vi "_LecturaLOG_Datos_TDMS.vi"(11 "Path":path) -> ()   [LabVIEW 2018]
uses:
  TypeDefsTopside/Top Data.ctl
  Shared/Type Defs/ROV States.ctl
  TypeDefsSubsea/Modos Control.ctl
  TypeDefsTopside/DAQ Top Data.ctl
  TypeDefsTopside/User Data.ctl
  TypeDefsTopside/CI Data.ctl
  TypeDefsTopside/Surface Input Data.ctl
  TypeDefsTopside/Virtual User Interface Data.ctl
  TypeDefsTopside/Top Control.ctl
  TypeDefsSubsea/Sub Data.ctl
  TypeDefsSubsea/Sub Status.ctl
  Shared/Type Defs/SMP.ctl
  Shared/Type Defs/PWR.ctl
  Shared/Type Defs/Motor.ctl
  Shared/Type Defs/MotorNames.ctl
  Shared/Type Defs/SmartCard.ctl
  Shared/Type Defs/Box Names.ctl
  TypeDefsSubsea/Sub Control.ctl
  TypeDefsSubsea/ROV Outputs.ctl
  TypeDefsSubsea/Motor Control.ctl
  TypeDefsSubsea/Type Defs Subsea.lvlib
  TypeDefsTopside/Type Defs Topside.lvlib
panel:
  out "Progreso TopData":i32
  out "Progreso SubData":i32
  out "String":string
  out "subarray":T1[](array[typedef]) {"Control"."motor_ctrl_array"."sensor" format="%#.2f"; "Control"."motor_ctrl_array"."setpoint" format="%#.2f"; "Control"."dac_outputs" format="%#.2f"; "PWR"."motor_array"."motor_name" items=["Motor1", "Motor2", "Motor3", "Motor4", "Motor5", "Motor6"]}
  out "TppData":T14[](array[typedef]) {"Virtual CI"."pot_c2" step=0.1; "Virtual CI"."pot_c1" step=0.01; "Virtual CI"."pot_gen" step=1.0; "Virtual CI"."pot_l3" step=0.01; "Virtual CI"."pot_l2" step=0.01; "Virtual CI"."pot_l1" step=0.01; "Virtual CI"."pot_m6" step=0.01; "Virtual CI"."pot_m5" step=0.01; "Virtual CI"."pot_m4" step=0.01; "Virtual CI"."pot_m3" step=0.01; "Virtual CI"."pot_m2" step=0.01; "Virtual CI"."pot_m1" step=0.01; "DAQ"."vess_ahrs_"."yaw" format="%.2g"; "DAQ"."vess_ahrs_"."roll" format="%.2g"; "DAQ"."vess_ahrs_"."pitch" format="%.2g"; "DAQ"."usbl_"."z" format="%.7g"; "DAQ"."usbl_"."y" format="%.7g"; "DAQ"."usbl_"."x" format="%.7g"; "DAQ"."gps_"."alt" format="%.7g"; "DAQ"."gps_"."lon" format="%.7g"; "DAQ"."gps_"."lat" format="%.7g"}
  in  "index":i32
  out "Waveform Graph":waveform(dbl)[](graph)
  out "Fecha y hora fin":timestamp
  out "Fecha y hora Inicio":timestamp
  out "error out":errorcluster
  out "Total datos":i32
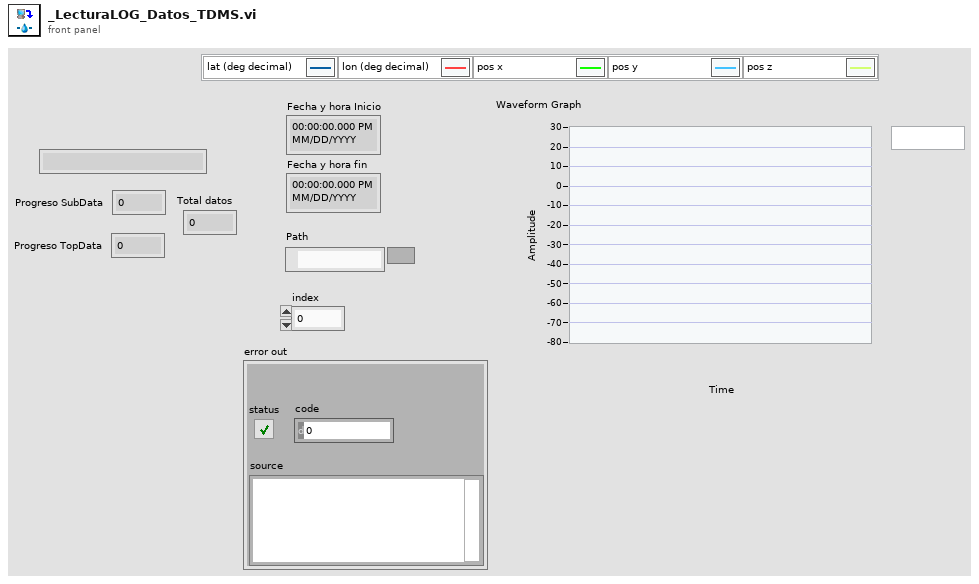
[diagram p1: front panel]
types:
  T1 = typedef "Type Defs Subsea.lvlib/Sub Data.ctl" = cluster{"Status":T2, "AHRS":cluster{"id_sensor":u32, "id_daq":u64, "pitch":dbl, "roll":dbl, "heading":dbl, "accel_x":dbl, "accel_y":dbl, "accel_z":dbl, "gyr_x":dbl, "gyr_y":dbl, "gyr_z":dbl, "mag_x":dbl, "mag_y":dbl, "mag_z":dbl, "acquisition_time":timestamp}, "CTD":cluster{"id_sensor":u32, "id_daq":u64, "pressure":dbl, "temperature":dbl, "conductivity":dbl, "density":dbl, "salinity":dbl, "speed_of_sound":dbl, "depth":dbl, "acquisition_time":timestamp}, "ALTIMETER":cluster{"id_sensor":u32, "id_daq":u64, "altitude":dbl, "acquisition_time":timestamp}, "SMP":T4, "PWR":T5, "SC_PWR":T8, "SC_CPU":T8, "SC_SMP":T8, "Control":T10}
  T2 = typedef "Type Defs Subsea.lvlib/Sub Status.ctl" = cluster{"id_sensor":u32, "id_daq":u32, "sub_ind":bool, "sample_time":i64, "sc_ind":bool[], "rov_states":T3, "acquisition_time":timestamp}
  T3 = typedef "Type Defs Subsea.lvlib/ROV States.ctl" = enum16{"INIT", "IDLE", "TEST", "RUN", "EMERGENCY", "EXIT"}
  T4 = typedef "Type Defs Subsea.lvlib/SMP.ctl" = cluster{"id_sensor":u32, "id_daq":u64, "liquid_smp1":bool, "liquid_smp2":bool, "liquid_smp3":bool, "liquid_smp4":bool, "solid_smp1":bool, "solid_smp2":bool, "supply_12v":bool, "motor_signal1":dbl, "motor_signal2":dbl, "cur_liq_1":dbl, "cur_liq_2":dbl, "acquisition_time":timestamp}
  T5 = typedef "Type Defs Topside.lvlib/PWR.ctl" = cluster{"id_sensor":u32, "id_daq":u64, "ac_status":bool, "voltage_hvdc":dbl, "current_hvdc":dbl, "motor_array":T6[], "light1":dbl, "light2":dbl, "light_sphere":dbl, "voltage_l1_l2":dbl, "voltage_l2_l3":dbl, "voltage_l1_l3":dbl, "current_l1":dbl, "current_l2":dbl, "current_l3":dbl, "current_lights":dbl, "temp_ac_filter":dbl, "acquisition_time":timestamp}
  T6 = typedef "Type Defs Subsea.lvlib/Motor.ctl" = cluster{"motor_name":T7, "status":bool, "ctrl_signal":dbl, "current":dbl, "speed":dbl}
  T7 = typedef "Type Defs Subsea.lvlib/MotorNames.ctl" = u16
  T8 = typedef "Type Defs Subsea.lvlib/SmartCard.ctl" = cluster{"id_sensor":u32, "id_daq":u64, "box_name":T9, "mode":enum16{"OFF", "STANDBY", "TESTING", "RUN", "EMERGENCY"}, "stat":dbl, "lps":dbl, "controller":dbl, "voltage":dbl, "current":dbl, "temperature":dbl, "humidity":dbl, "leak":dbl, "pressure":dbl, "acquisition_time":timestamp}
  T9 = typedef "Type Defs Subsea.lvlib/Box Names.ctl" = enum16{"PWR", "CPU", "SMP"}
  T10 = typedef "Type Defs Subsea.lvlib/Sub Control.ctl" = cluster{"id_sensor":u32, "id_daq":u64, "ctrl_state":T11, "rov_output":T12, "dac_outputs":dbl[], "motor_ctrl_array":T13[], "in_range":bool[], "acquisition_time":timestamp}
  T11 = typedef "Type Defs Subsea.lvlib/Modos Control.ctl" = enum16{"Manual", "Profundidad", "Altitud", "Rumbo", "P+R"}
  T12 = typedef "Type Defs Subsea.lvlib/ROV Outputs.ctl" = cluster{"x":dbl, "y":dbl, "z":dbl, "yaw":dbl}
  T13 = typedef "Type Defs Subsea.lvlib/Motor Control.ctl" = cluster{"setpoint":dbl, "sensor":dbl}
  T14 = typedef "Type Defs Topside.lvlib/Top Data.ctl" = cluster{"Status":cluster{"id_sensor":u32, "Ind.":bool, "sample time":u32, "rov_states":T3, "acquisition_time":timestamp, "modo_ctrl":T11}, "DAQ":T15, "User Data":T16, "Virtual CI":T19, "Control":T20}
  T15 = typedef "Type Defs Topside.lvlib/DAQ Top Data.ctl" = cluster{"id_daq":u32, "id_sensor":u32, "gps_":cluster{"lat":dbl, "lon":dbl, "alt":dbl}, "usbl_":cluster{"x":dbl, "y":dbl, "z":dbl}, "vess_ahrs_":cluster{"pitch":dbl, "roll":dbl, "yaw":dbl}, "acquisition_time":timestamp}
  T16 = typedef "Type Defs Topside.lvlib/User Data.ctl" = cluster{"id_sensor":u32, "id_daq":u64, "ci_habilitada":bool, "acquisition_time":timestamp, "CI Data":T17, "Surface Data":T18}
  T17 = typedef "Type Defs Topside.lvlib/CI Data.ctl" = cluster{"joy_1x":dbl, "joy_1y":dbl, "joy_1z":dbl, "joy_1thumb":dbl, "joy_1botIzq":u8, "joy_1botder":u8, "joy_1gatillo":u8, "modo_1bot":u8, "modo_2bot":u8, "modo_3bot":u8, "modo_4bot":u8, "pot":dbl, "enc":dbl, "joy_2x":dbl, "joy_2y":dbl, "joy_2z":dbl, "joy_2bot":u8, "botella_1bot":u8, "botella_2bot":u8, "botella_3bot":u8, "botella_4bot":u8, "corer_1bot":u8, "corer_2bot":u8, "a_in":dbl, "dio1":u8, "dio2":u8, "dio3":u8, "ci_acc_x":dbl, "ci_acc_y":dbl, "ci_acc_z":dbl}
  T18 = typedef "Type Defs Topside.lvlib/Surface Input Data.ctl" = cluster{"modo_1ind":u8, "modo_2ind":u8, "modo_3ind":u8, "modo_4ind":u8, "botella_1ind":u8, "botella_2ind":u8, "botella_3ind":u8, "botella_4ind":u8, "corer_1ind":u8, "corer_2ind":u8, "lars_vel":dbl, "lars_fwd":u8, "lars_rev":u8}
  T19 = typedef "Type Defs Topside.lvlib/Virtual User Interface Data.ctl" = cluster{"id_sensor":u32, "id_daq":u64, "bus_260v":bool, "m_6":bool, "m_5":bool, "m_2":bool, "m_1":bool, "m_4":bool, "m_3":bool, "luz_1":bool, "luz_2":bool, "luz_3":bool, "pot_m1":dbl, "pot_m2":dbl, "pot_m3":dbl, "pot_m4":dbl, "pot_m5":dbl, "pot_m6":dbl, "pot_l1":dbl, "pot_l2":dbl, "pot_l3":dbl, "pot_gen":dbl, "fuente_muestras":bool, "bot_1":bool, "bot_2":bool, "bot_3":bool, "bot_4":bool, "corer_1":bool, "corer_2":bool, "pot_c1":dbl, "pot_c2":dbl, "virtual_ci":bool, "acquisition_time":timestamp}
  T20 = typedef "Type Defs Topside.lvlib/Top Control.ctl" = cluster{"depth_PID":cluster{"Kp":dbl, "Ti":dbl, "Td":dbl}, "heading_PID":cluster{"Kp":dbl, "Ti":dbl, "Td":dbl}, "altitude_PID":cluster{"Kp":dbl, "Ti":dbl, "Td":dbl}, "depth_sp":dbl, "heading_sp":dbl, "altitude_sp":dbl, "m_PID_en":bool, "PID_reset":bool, "acquisition_time":timestamp, "motor_PID":cluster{"Kp":dbl, "Ti":dbl, "Td":dbl}, "m1_lo":dbl, "m1_hi":dbl, "m1_en":bool, "m2_lo":dbl, "m2_hi":dbl, "m2_en":bool, "m3_lo":dbl, "m3_hi":dbl, "m3_en":bool, "m4_lo":dbl, "m4_hi":dbl, "m4_en":bool, "m5_lo":dbl, "m5_hi":dbl, "m5_en":bool, "m6_lo":dbl, "m6_hi":dbl, "m6_en":bool, "modo_ctrl":T11}
  T21 = enum16{"open", "open or create", "create or replace", "create", "open (read-only)"}
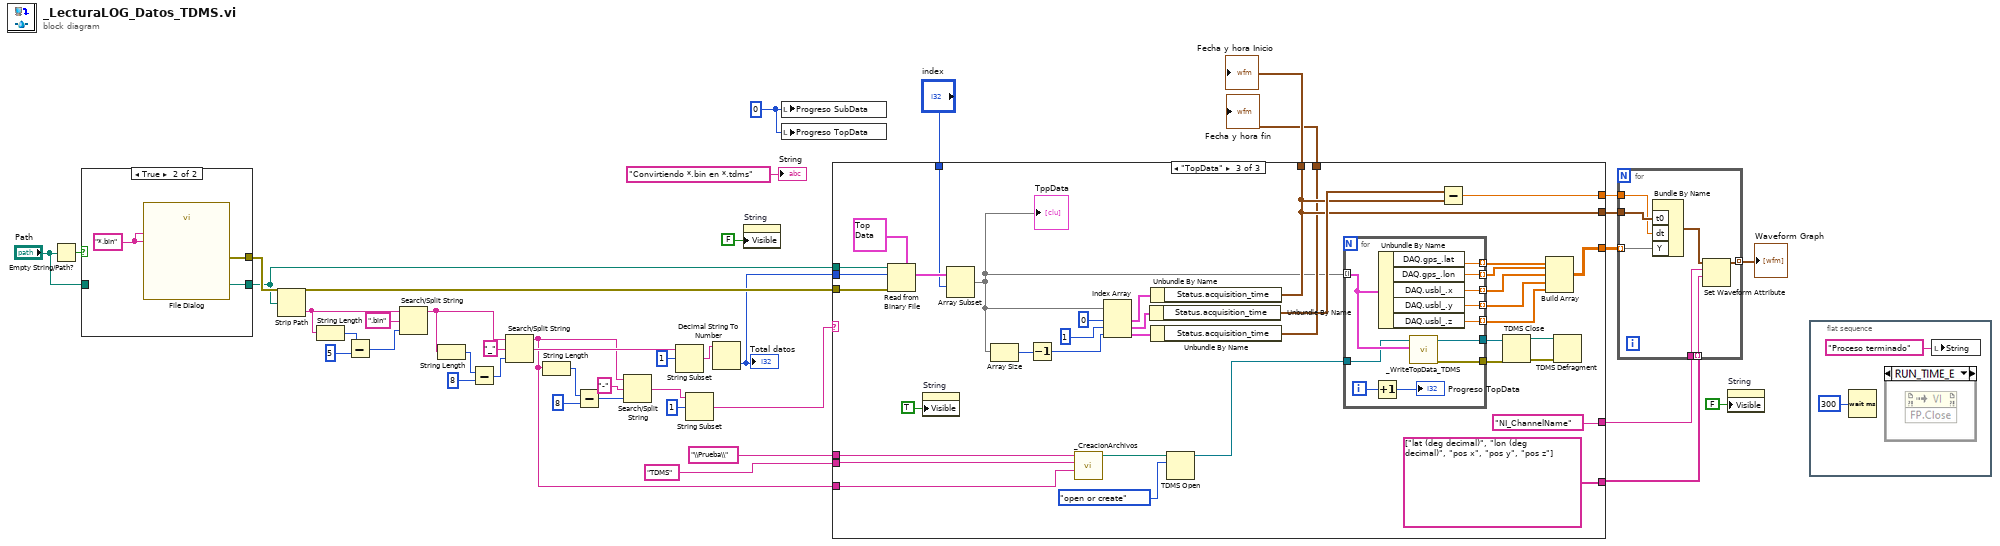
[diagram p0: block diagram]
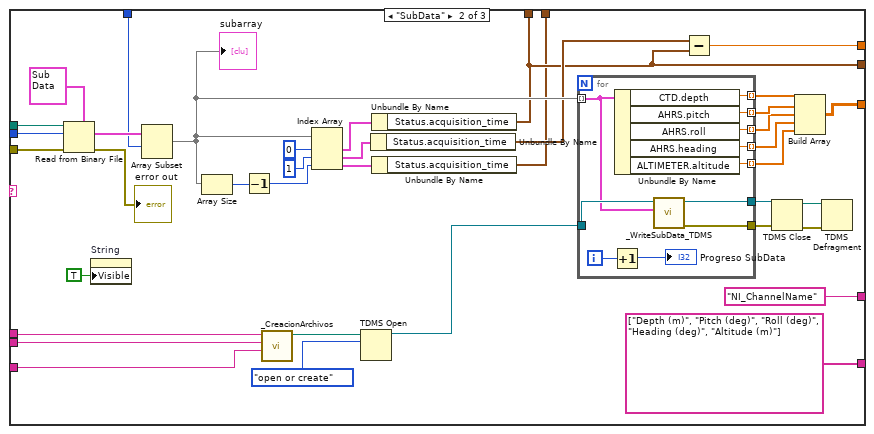
[diagram p4: hidden frame]
diagram:
  w2 = 0 ("Progreso SubData")
  n1 = Empty String/Path?(string/path="Path") -> (empty?=w19:bool)
  n2 = case shown="True" w19 {
    tunnel: [_ w45] -> w41
    tunnel: [w42 w44] -> w40
    tunnel: "Path" -> [w42 _]
    frame False {
    }
    frame True {
      w43 = "*.bin" ("pattern (all files)")
      n3 = call "File Dialog"("pattern (all files)"=w43, "pattern label"=w43) -> ("selected path"=w44:path, "error out"=w45:errorcluster)  [unwired: 10 in, 2 out]
    }
  }
  n4 = Strip Path(path=w40) -> (name=w39:string)  [unwired: 1 out]
  n5 = String Length(string=w39) -> (length=w38:i32)
  n6 = Subtract(x=w38, y=5) -> (x-y=w36:i32)
  n7 = Search/Split String(string=w39, search string/char (-)=".bin", offset (0)=w36) -> (substring before match=w34:string)  [unwired: 2 out]
  n8 = String Length(string=w34) -> (length=w33:i32)
  n9 = Subtract(x=w33, y=8) -> (x-y=w31:i32)
  n10 = Search/Split String(string=w34, search string/char (-)="_", offset (0)=w31) -> (substring before match=w7:string, match + rest of string=w29:string)  [unwired: 1 out]
  n11 = String Length(string=w7) -> (length=w25:i32)
  n12 = Subtract(x=w25, y=8) -> (x-y=w24:i32)
  n13 = Search/Split String(string=w7, search string/char (-)="-", offset (0)=w24) -> (match + rest of string=w21:string)  [unwired: 2 out]
  n14 = String Subset(string=w29, offset (0)=1) -> (substring=w22:string)  [unwired: 1 in]
  n15 = String Subset(string=w21, offset (0)=1) -> (substring=w20:string)  [unwired: 1 in]
  n16 = Decimal String To Number(string=w22) -> (number=w1:i32)  [unwired: 2 in, 1 out]
  "Total datos" <- w1
  n17 = property on="String" class="Str"("Visible"=FALSE) -> ()  [unwired: 2 in, 2 out]
  n18 = local write "Progreso SubData"(w2) -> ()
  n19 = local write "Progreso TopData"(w2) -> ()
  n20 = case shown="\"TopData\"" w20 {
    tunnel: w41 -> [_ w83 w131]
    tunnel: w40 -> [_ w82 w130]
    tunnel: w1 -> [_ w81 w129]
    tunnel: [_ w60 w118] -> w16
    tunnel: [_ "NI_ChannelName" ("name") "NI_ChannelName" ("name")] -> w3
    tunnel: [_ w63 w117] -> w15
    tunnel: [_ string[] ["Depth (m)", "Pitch (deg)", "Roll (deg)", "Heading (deg)", "Altitude (m)"] string[] ["lat (deg decimal)", "lon (deg decimal)", "pos x", "pos y", "pos z"]] -> w14
    tunnel: [_ w61 w96] -> w13
    tunnel: [_ w60 w118] -> w12
    tunnel: [_ w59 w116] -> w11
    tunnel: "index" -> [_ w58 w123]
    tunnel: "TDMS" ("Nombre_mision") -> [_ w52 w100]
    tunnel: "\\Prueba\\" ("Carpeta") -> [_ w51 w101]
    tunnel: w7 -> [_ w49 w97]
    frame Default {
    }
    frame "SubData" {
      n21 = Read from Binary File(5:T1 {"Status"={"id_sensor"=0, "id_daq"=0, "sub_ind"=FALSE, "sample_time"=0, "sc_ind"=[FALSE, FALSE, FALSE], "rov_states"=enum."INIT", "acquisition_time"=timestamp(0 s since 1904-01-01)}, "AHRS"={"id_sensor"=0, "id_daq"=0, "pitch"=0.0, "roll"=0.0, "heading"=0.0, "accel_x"=0.0, "accel_y"=0.0, "accel_z"=0.0, "gyr_x"=0.0, "gyr_y"=0.0, "gyr_z"=0.0, "mag_x"=0.0, "mag_y"=0.0, "mag_z"=0.0, "acquisition_time"=timestamp(0 s since 1904-01-01)}, "CTD"={"id_sensor"=0, "id_daq"=0, "pressure"=0.0, "temperature"=0.0, "conductivity"=0.0, "density"=0.0, "salinity"=0.0, "speed_of_sound"=0.0, "depth"=0.0, "acquisition_time"=timestamp(0 s since 1904-01-01)}, "ALTIMETER"={"id_sensor"=0, "id_daq"=0, "altitude"=0.0, "acquisition_time"=timestamp(0 s since 1904-01-01)}, "SMP"={"id_sensor"=0, "id_daq"=0, "liquid_smp1"=FALSE, "liquid_smp2"=FALSE, "liquid_smp3"=FALSE, "liquid_smp4"=FALSE, "solid_smp1"=FALSE, "solid_smp2"=FALSE, "supply_12v"=FALSE, "motor_signal1"=0.0, "motor_signal2"=0.0, "cur_liq_1"=0.0, "cur_liq_2"=0.0, "acquisition_time"=timestamp(0 s since 1904-01-01)}, "PWR"={"id_sensor"=0, "id_daq"=0, "ac_status"=FALSE, "voltage_hvdc"=0.0, "current_hvdc"=0.0, "motor_array"=[], "light1"=0.0, "light2"=0.0, "light_sphere"=0.0, "voltage_l1_l2"=0.0, "voltage_l2_l3"=0.0, "voltage_l1_l3"=0.0, "current_l1"=0.0, "current_l2"=0.0, "current_l3"=0.0, "current_lights"=0.0, "temp_ac_filter"=0.0, "acquisition_time"=timestamp(0 s since 1904-01-01)}, "SC_PWR"={"id_sensor"=0, "id_daq"=0, "box_name"=enum."PWR", "mode"=enum."OFF", "stat"=0.0, "lps"=0.0, "controller"=0.0, "voltage"=0.0, "current"=0.0, "temperature"=0.0, "humidity"=0.0, "leak"=0.0, "pressure"=0.0, "acquisition_time"=timestamp(0 s since 1904-01-01)}, "SC_CPU"={"id_sensor"=0, "id_daq"=0, "box_name"=enum."PWR", "mode"=enum."OFF", "stat"=0.0, "lps"=0.0, "controller"=0.0, "voltage"=0.0, "current"=0.0, "temperature"=0.0, "humidity"=0.0, "leak"=0.0, "pressure"=0.0, "acquisition_time"=timestamp(0 s since 1904-01-01)}, "SC_SMP"={"id_sensor"=0, "id_daq"=0, "box_name"=enum."PWR", "mode"=enum."OFF", "stat"=0.0, "lps"=0.0, "controller"=0.0, "voltage"=0.0, "current"=0.0, "temperature"=0.0, "humidity"=0.0, "leak"=0.0, "pressure"=0.0, "acquisition_time"=timestamp(0 s since 1904-01-01)}, "Control"={"id_sensor"=0, "id_daq"=0, "ctrl_state"=enum."Manual", "rov_output"={"x"=0.0, "y"=0.0, "z"=0.0, "yaw"=0.0}, "dac_outputs"=[], "motor_ctrl_array"=[], "in_range"=[], "acquisition_time"=timestamp(0 s since 1904-01-01)}} ("Sub Data"), 8:w83, 10:w81, 11:w82) -> (0:→"error out":errorcluster, 2:w79:T1[])  [unwired: 2 in, 2 out]
      n22 = property on="String" class="Str"("Visible"=TRUE) -> ()  [unwired: 2 in, 2 out]
      n23 = Array Subset(array=w79, index=w58) -> (w75:T1[])  [unwired: 1 in]
      "subarray" <- w75
      n24 = Array Size(array=w75) -> (size(s)=w78:i32)
      n25 = Decrement(x=w78) -> (x-1=w74:i32)
      n26 = call "_CreacionArchivos.vi"("Tipo_Data"=w49, "Nombre_mision"=w52, "Carpeta"=w51) -> ("appended path"=w54:path)  [unwired: 8 in]
      n27 = Index Array(array=w75, index #1=0 ("index"), index #2=1 ("index"), index #3=w74) -> (element #1=w76:T1, element #2=w71:T1, element #3=w72:T1)
      n28 = TDMS Open(10:T21."open or create" ("operation (0:open)"), 11:w54) -> (3:w50:refnum<k34>)  [unwired: 5 in, 1 out]
      n29 = Unbundle By Name(w71) -> ("Status.acquisition_time"=w70:timestamp)
      n30 = Unbundle By Name(w76) -> ("Status.acquisition_time"=w60:timestamp)
      n31 = Unbundle By Name(w72) -> ("Status.acquisition_time"=w59:timestamp)
      n32 = for {
        tunnel: w75 -> [w86] mode=indexing
        tunnel: [w94] -> w69 mode=indexing
        tunnel: [w93] -> w68 mode=indexing
        tunnel: [w92] -> w67 mode=indexing
        tunnel: [w91] -> w66 mode=indexing
        tunnel: [w90] -> w65 mode=indexing
        tunnel: w50 -> [w89]
        tunnel: [w87] -> w56
        tunnel: [w88] -> w55
        i -> [w85]
        n33 = Increment(x=w85) -> (x+1=→"Progreso SubData":i32)
        n34 = Unbundle By Name(w86) -> ("CTD.depth"=w94:dbl, "AHRS.pitch"=w93:dbl, "AHRS.roll"=w92:dbl, "AHRS.heading"=w91:dbl, "ALTIMETER.altitude"=w90:dbl)
        n35 = call "_WriteSubData_TDMS.vi"("Sub Data in"=w86, "Refnum in"=w89) -> ("error out"=w87:errorcluster, "Refnum out"=w88:refnum<k34>)  [unwired: 8 in]
      }
      n36 = Subtract(x=w70, y=w60) -> (x-y=w63:dbl)
      n37 = TDMS Close(8:w56, 11:w55) -> (0:w48:errorcluster, 3:w47:path)
      n38 = Build Array(w69, w68, w67, w66, w65) -> (w61:dbl[][])
      n39 = TDMS Defragment(4:w48, 7:w47) -> ()  [unwired: 1 out]
    }
    frame "TopData" {
      n40 = Read from Binary File(5:T14 {"Status"={"id_sensor"=1, "Ind."=FALSE, "sample time"=0, "rov_states"=enum."INIT", "acquisition_time"=timestamp(0 s since 1904-01-01), "modo_ctrl"=enum."Manual"}, "DAQ"={"id_daq"=0, "id_sensor"=0, "gps_"={"lat"=0.0, "lon"=0.0, "alt"=0.0}, "usbl_"={"x"=0.0, "y"=0.0, "z"=0.0}, "vess_ahrs_"={"pitch"=0.0, "roll"=0.0, "yaw"=0.0}, "acquisition_time"=timestamp(0 s since 1904-01-01)}, "User Data"={"id_sensor"=0, "id_daq"=0, "ci_habilitada"=FALSE, "acquisition_time"=timestamp(0 s since 1904-01-01), "CI Data"={"joy_1x"=2.5, "joy_1y"=2.5, "joy_1z"=2.5, "joy_1thumb"=2.5, "joy_1botIzq"=0, "joy_1botder"=0, "joy_1gatillo"=0, "modo_1bot"=0, "modo_2bot"=0, "modo_3bot"=0, "modo_4bot"=0, "pot"=0.0, "enc"=0.0, "joy_2x"=0.0, "joy_2y"=0.0, "joy_2z"=0.0, "joy_2bot"=0, "botella_1bot"=0, "botella_2bot"=0, "botella_3bot"=0, "botella_4bot"=0, "corer_1bot"=0, "corer_2bot"=0, "a_in"=0.0, "dio1"=0, "dio2"=0, "dio3"=0, "ci_acc_x"=0.0, "ci_acc_y"=0.0, "ci_acc_z"=0.0}, "Surface Data"={"modo_1ind"=0, "modo_2ind"=0, "modo_3ind"=0, "modo_4ind"=0, "botella_1ind"=0, "botella_2ind"=0, "botella_3ind"=0, "botella_4ind"=0, "corer_1ind"=0, "corer_2ind"=0, "lars_vel"=0.0, "lars_fwd"=0, "lars_rev"=0}}, "Virtual CI"={"id_sensor"=0, "id_daq"=0, "bus_260v"=FALSE, "m_6"=FALSE, "m_5"=FALSE, "m_2"=FALSE, "m_1"=FALSE, "m_4"=FALSE, "m_3"=FALSE, "luz_1"=FALSE, "luz_2"=FALSE, "luz_3"=FALSE, "pot_m1"=0.0, "pot_m2"=0.0, "pot_m3"=0.0, "pot_m4"=0.0, "pot_m5"=0.0, "pot_m6"=0.0, "pot_l1"=0.0, "pot_l2"=0.0, "pot_l3"=0.0, "pot_gen"=0.0, "fuente_muestras"=FALSE, "bot_1"=FALSE, "bot_2"=FALSE, "bot_3"=FALSE, "bot_4"=FALSE, "corer_1"=FALSE, "corer_2"=FALSE, "pot_c1"=0.0, "pot_c2"=0.0, "virtual_ci"=FALSE, "acquisition_time"=timestamp(0 s since 1904-01-01)}, "Control"={"depth_PID"={"Kp"=0.0, "Ti"=0.03, "Td"=0.001}, "heading_PID"={"Kp"=0.05, "Ti"=0.03, "Td"=0.001}, "altitude_PID"={"Kp"=0.05, "Ti"=0.03, "Td"=0.001}, "depth_sp"=0.0, "heading_sp"=0.0, "altitude_sp"=0.0, "m_PID_en"=FALSE, "PID_reset"=FALSE, "acquisition_time"=timestamp(0 s since 1904-01-01), "motor_PID"={"Kp"=0.05, "Ti"=0.03, "Td"=0.001}, "m1_lo"=0.0, "m1_hi"=0.0, "m1_en"=TRUE, "m2_lo"=0.0, "m2_hi"=0.0, "m2_en"=TRUE, "m3_lo"=0.0, "m3_hi"=0.0, "m3_en"=TRUE, "m4_lo"=0.0, "m4_hi"=5.0, "m4_en"=TRUE, "m5_lo"=-5.0, "m5_hi"=5.0, "m5_en"=TRUE, "m6_lo"=-5.0, "m6_hi"=5.0, "m6_en"=TRUE, "modo_ctrl"=enum."Manual"}} ("Top Data"), 8:w131, 10:w129, 11:w130) -> (2:w124:T14[])  [unwired: 2 in, 3 out]
      n41 = property on="String" class="Str"("Visible"=TRUE) -> ()  [unwired: 2 in, 2 out]
      n42 = Array Subset(array=w124, index=w123) -> (w108:T14[])  [unwired: 1 in]
      "TppData" <- w108
      n43 = Array Size(array=w108) -> (size(s)=w128:i32)
      n44 = Decrement(x=w128) -> (x-1=w127:i32)
      n45 = call "_CreacionArchivos.vi"("Tipo_Data"=w97, "Nombre_mision"=w100, "Carpeta"=w101) -> ("appended path"=w104:path)  [unwired: 8 in]
      n46 = Index Array(array=w108, index #1=0 ("index"), index #2=1 ("index"), index #3=w127) -> (element #1=w122:T14, element #2=w121:T14, element #3=w120:T14)
      n47 = Unbundle By Name(w121) -> ("Status.acquisition_time"=w119:timestamp)
      n48 = Unbundle By Name(w122) -> ("Status.acquisition_time"=w118:timestamp)
      n49 = Unbundle By Name(w120) -> ("Status.acquisition_time"=w116:timestamp)
      n50 = TDMS Open(10:T21."open or create" ("operation (0:open)"), 11:w104) -> (3:w102:refnum<k34>)  [unwired: 5 in, 1 out]
      n51 = for {
        tunnel: w108 -> [w137] mode=indexing
        tunnel: [w142] -> w113 mode=indexing
        tunnel: [w141] -> w112 mode=indexing
        tunnel: [w140] -> w111 mode=indexing
        tunnel: [w139] -> w110 mode=indexing
        tunnel: [w138] -> w109 mode=indexing
        tunnel: w102 -> [w136]
        tunnel: [w134] -> w106
        tunnel: [w135] -> w105
        i -> [w133]
        n52 = Increment(x=w133) -> (x+1=→"Progreso TopData":i32)
        n53 = Unbundle By Name(w137) -> ("DAQ.gps_.lat"=w142:dbl, "DAQ.gps_.lon"=w141:dbl, "DAQ.usbl_.x"=w140:dbl, "DAQ.usbl_.y"=w139:dbl, "DAQ.usbl_.z"=w138:dbl)
        n54 = call "_WriteTopData_TDMS.vi"("Top Data in"=w137, "Refnum in"=w136) -> ("error out"=w134:errorcluster, "Refnum out"=w135:refnum<k34>)  [unwired: 8 in]
      }
      n55 = Subtract(x=w119, y=w118) -> (x-y=w117:dbl)
      n56 = TDMS Close(8:w106, 11:w105) -> (0:w98:errorcluster, 3:w99:path)
      n57 = Build Array(w113, w112, w111, w110, w109) -> (w96:dbl[][])
      n58 = TDMS Defragment(4:w98, 7:w99) -> ()  [unwired: 1 out]
    }
  }
  "Fecha y hora Inicio" <- w12
  "Fecha y hora fin" <- w11
  n59 = for {
    tunnel: w16 -> [w149]
    tunnel: w3 -> [w148]
    tunnel: w15 -> [w147]
    tunnel: w14 -> [w145] mode=indexing
    tunnel: [w144] -> w17 mode=indexing
    tunnel: w13 -> [w143] mode=indexing
    n60 = Bundle By Name("t0"=w149, "dt"=w147, "Y"=w143) -> (w146:waveform(dbl))  [unwired: 1 in]
    n61 = Set Waveform Attribute(5:w145, 6:w148, 7:w146) -> (3:w144:waveform(dbl))  [unwired: 1 in, 2 out]
  }
  "Waveform Graph" <- w17
  n62 = property on="String" class="Str"("Visible"=FALSE) -> ()  [unwired: 2 in, 2 out]
  n63 = flat-sequence {
    frame #0 {
      n64 = Wait (ms)(milliseconds to wait=u32 300) -> ()  [unwired: 1 out]
      n65 = local write "String"("Proceso terminado" ("String")) -> ()
    }
  }
  "String" <- "Convirtiendo *.bin en *.tdms" ("String")
